vi "PrepareChannels_htsp.vi"(10 "Sampling Rate (Hz)":dbl=100000.0) -> (0 "DO error out":errorcluster, 1 "DO task out":refnum<k21>, 2 "AO error out":errorcluster, 3 "AO task out":refnum<k21>, 5 "Pulse":dbl[](array[numeric]), 7 "Pulse length":i32)   [LabVIEW 2015]
uses:
  <vilib>/DAQmx/create/channels.llb/DAQmx Create Channel (AO-Voltage-Basic).vi
  <vilib>/DAQmx/configure/timing.llb/DAQmx Timing (Sample Clock).vi
  <vilib>/DAQmx/create/channels.llb/DAQmx Create Channel (DO-Digital Output).vi
panel:
  in  "AO Timing channel":tag
  in  "DO Physical channels":tag="Dev1/port0/line0"
  in  "Amplitude (Volts)":dbl=1.0
  out "Waveform Graph":waveform(dbl)(graph)
  in  "Num Pulses":u32=1 min=1
  in  "Pulse Width (ms)":dbl=0.09
  in  "Pulse Type":enum16{"Monophasic", "Biphasic"}(ring)=enum."Biphasic"
  in  "AO Physical channels":tag="Dev1/ao0"
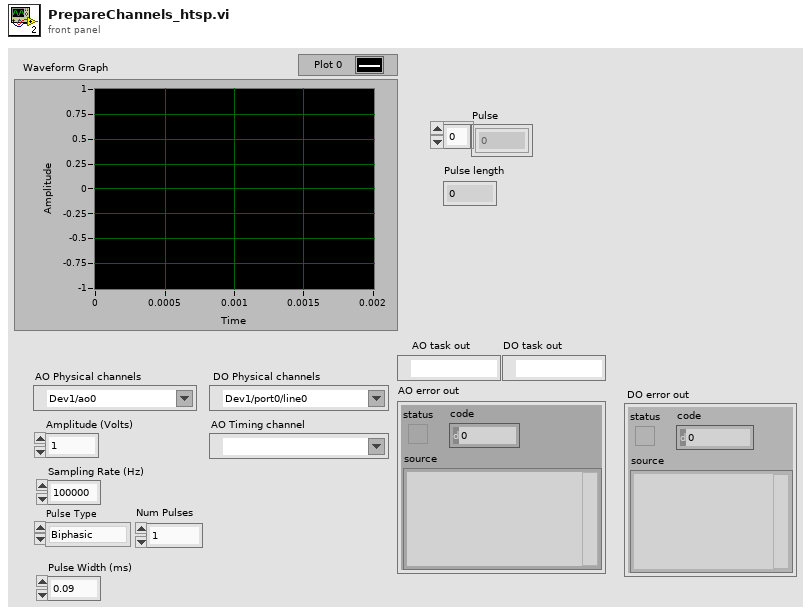
[diagram p1: front panel]
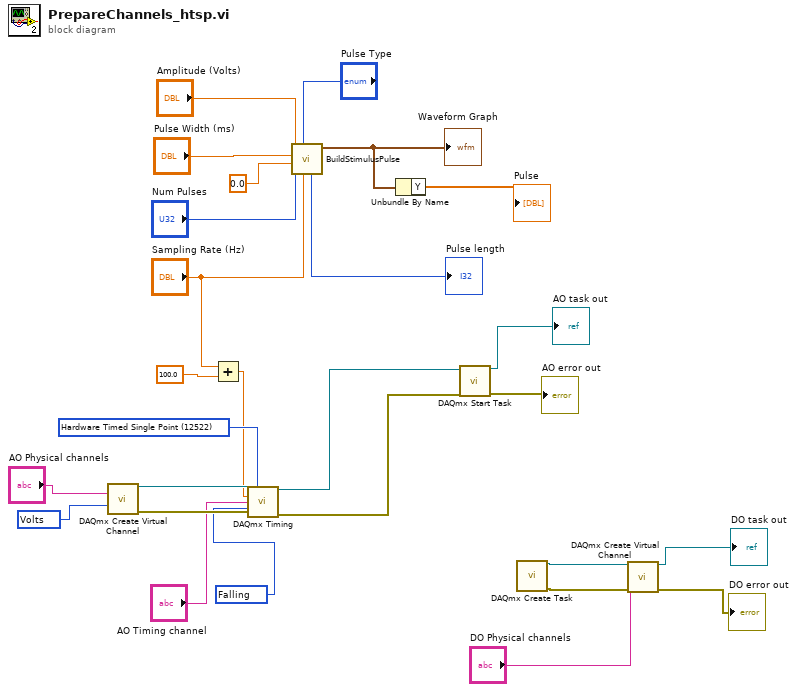
[diagram p0: block diagram]
diagram:
  w1 = 10171 items=["Rising"=10280, "Falling"=10171] ("active edge")
  w20 = 12522 items=["Finite Samples"=10178, "Continuous Samples"=10123, "Hardware Timed Single Point"=12522] ("sample mode")
  w27 = 10348 items=["Volts"=10348, "From Custom Scale"=10065] ("units")
  n1 = call-poly <vilib>:"DAQmx Create Virtual Channel.vi"("physical channels"="AO Physical channels", "units"=w27) -> ("task out"=w18:refnum<k21>, "error out"=w17:errorcluster)  [unwired: 12 in]
  n2 = Add(x="Sampling Rate (Hz)", y=100.0) -> (x+y=w2:dbl)
  n3 = call-poly <vilib>:"DAQmx Timing.vi"("task/channels in"=w18, "sample mode"=w20, "rate"=w2, "source"="AO Timing channel", "active edge"=w1, "error in"=w17) -> ("task out"=w11:refnum<k21>, "error out"=w10:errorcluster)  [unwired: 8 in]
  n4 = call "BuildStimulusPulse.vi"("Sampling Rate (Hz)"="Sampling Rate (Hz)", "Pulse Type"="Pulse Type", "Num Pulses"="Num Pulses", "Inter-Pulse Interval (ms)"=0.0, "Pulse Width (ms)"="Pulse Width (ms)", "Amplitude (Volts)"="Amplitude (Volts)") -> ("Waveform Out"=w7:waveform(dbl), "Final Array Size"=→"Pulse length":i32)  [unwired: 3 in, 1 out]
  "Waveform Graph" <- w7
  n5 = Unbundle By Name(w7) -> ("Y"=→"Pulse":dbl[])
  n6 = call <vilib>:"DAQmx Start Task.vi"("task/channels in"=w11, "error in"=w10) -> ("task out"=→"AO task out":refnum<k21>, "error out"=→"AO error out":errorcluster)  [unwired: 12 in]
  n7 = call <vilib>:"DAQmx Create Task.vi"() -> ("task out"=w15:refnum<k21>, "error out"=w14:errorcluster)  [unwired: 14 in]
  n8 = call-poly <vilib>:"DAQmx Create Virtual Channel.vi"("task in"=w15, "lines"="DO Physical channels", "error in"=w14) -> ("task out"=→"DO task out":refnum<k21>, "error out"=→"DO error out":errorcluster)  [unwired: 11 in]
